vi "Is Interface Or LabVIEW Object.vi"(10 "LabVIEW Object":refnum<class>) -> (2 "Is Interface Or LabVIEW Object":bool)   [LabVIEW 2017, in "Composition.lvlib"]
doc: "Checks if the provided object is an interface or LabVIEW Object."
uses:
  Composition.lvlib
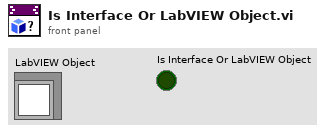
[diagram p1: front panel]
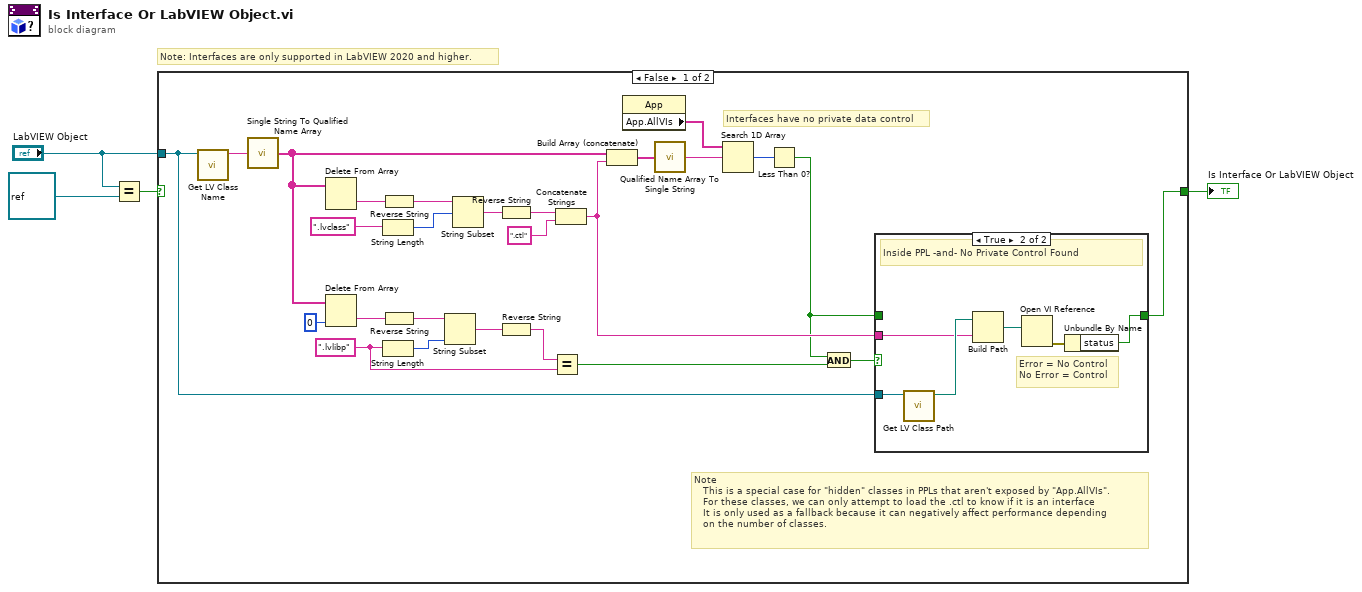
[diagram p0: block diagram]
diagram:
  # "Note: Interfaces are only supported in LabVIEW 2020 and higher."
  n1 = Equal?(x="LabVIEW Object", y=refnum<class> refnum) -> (x = y?=w3:bool)
  n2 = case shown="False" w3 {
    selector: w3 -> [_ w38]
    tunnel: "LabVIEW Object" -> [w10 _]
    tunnel: [w5 w38] -> w4
    frame False {
      w11 = ".lvlibp"
      # "Note\n   This is a special case for \"hidden\" classes in PPLs that aren't exposed by \"App.AllVIs\".\n   For these classes, we can only attempt to load the .ctl to know if it is an interface\n   It is only used as a fallback because it can negatively affect performance depending\n   on the number of classes."
      # "Interfaces have no private data control"
      n3 = call <vilib>:"Get LV Class Name.vi"("object"=w10) -> ("class name"=w26:string)  [unwired: 9 in, 1 out]
      n4 = call <vilib>:"Single String To Qualified Name Array.vi"("Fully Qualified String"=w26) -> ("Fully Qualified Array"=w18:string[])
      n5 = Delete From Array(array=w18) -> (deleted portion=w25:string)  [unwired: 2 in, 1 out]
      n6 = Delete From Array(array=w18, index=0) -> (deleted portion=w17:string)  [unwired: 1 in, 1 out]
      n7 = String Length(string=".lvclass") -> (length=w29:i32)
      n8 = String Length(string=w11) -> (length=w14:i32)
      n9 = Reverse String(1:w25) -> (0:w28:string)
      n10 = Reverse String(1:w17) -> (0:w15:string)
      n11 = String Subset(string=w15, length (rest)=w14) -> (substring=w13:string)  [unwired: 1 in]
      n12 = String Subset(string=w28, offset (0)=w29) -> (substring=w27:string)  [unwired: 1 in]
      n13 = Reverse String(1:w27) -> (0:w24:string)
      n14 = Reverse String(1:w13) -> (0:w12:string)
      n15 = Equal?(x=w12, y=w11) -> (x = y?=w8:bool)
      n16 = Concatenate Strings(w24, ".ctl" ("string")) -> (w9:string)
      n17 = Build Array (concatenate)(w18, w9) -> (w22:string[])
      n18 = property class="App"() -> ("App.AllVIs"=w20:string[])  [unwired: 2 in, 2 out]
      n19 = call <vilib>:"Qualified Name Array To Single String.vi"("Fully Qualified Array"=w22) -> ("Fully Qualified String"=w21:string)
      n20 = Search 1D Array(1D array=w20, element=w21) -> (index of element=w19:i32)  [unwired: 1 in]
      n21 = Less Than 0?(x=w19) -> (x < 0?=w6:bool)
      n22 = And(x=w6, y=w8) -> (x .and. y?=w7:bool)
      n23 = case shown="True" w7 {
        tunnel: w10 -> [_ w37]
        tunnel: w9 -> [_ w35]
        tunnel: [w31 w32] -> w5
        tunnel: w6 -> [w31 _]
        frame False {
          # "Private Control Found -or- Not PPL"
        }
        frame True {
          # "Error = No Control\nNo Error = Control"
          # "Inside PPL -and- No Private Control Found"
          n24 = call <vilib>:"Get LV Class Path.vi"("object"=w37) -> ("class path"=w36:path)  [unwired: 9 in, 1 out]
          n25 = Build Path(base path=w36, name or relative path=w35) -> (appended path=w34:path)
          n26 = Open VI Reference(vi path=w34) -> (error out=w33:errorcluster)  [unwired: 5 in, 1 out]
          n27 = Unbundle By Name(w33) -> ("status"=w32:bool)
        }
      }
    }
    frame True {
    }
  }
  "Is Interface Or LabVIEW Object" <- w4
